vi "Delete Item.vi"(0 "State In":T1={"Prompt"="Click to add", "Listbox"=refnum, "Required"={"Strings"=[], "Bottom"=FALSE, "Italic"=FALSE, "FG"=0, "BG"=16777215, "Bold"=FALSE}, "Items"=[], "Req'd"=[], "Events"={"Items Changed"=refnum, "List Changed"=refnum}, "Max Rows"=-1, "Default name"=""}, 7 "Delete at":i32) -> (4 "State Out":T1={"Prompt"="Click to add", "Listbox"=refnum, "Required"={"Strings"=[], "Bottom"=FALSE, "Italic"=FALSE, "FG"=0, "BG"=16777215, "Bold"=FALSE}, "Items"=[], "Req'd"=[], "Events"={"Items Changed"=refnum, "List Changed"=refnum}, "Max Rows"=-1, "Default name"=""})   [LabVIEW 2015, in "KListboxEx.xctl"]
uses:
  KListboxEx.xctl
  State.ctl
  Required.ctl
  Events.ctl
  Event Action.ctl
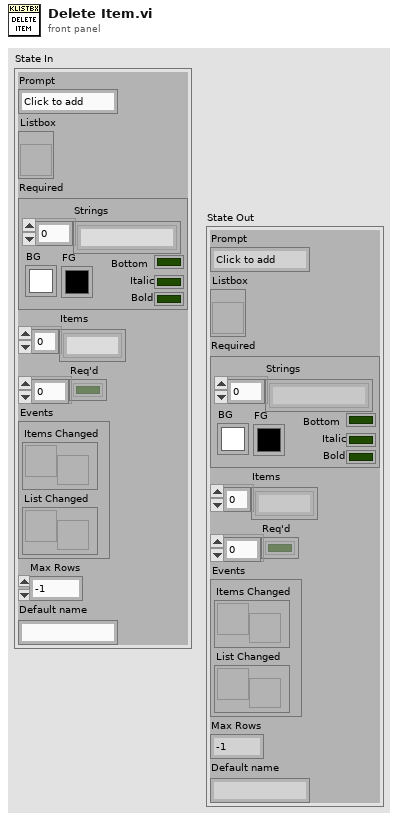
[diagram p1: front panel]
types:
  T1 = typedef "KListboxEx.xctl/State.ctl" = cluster{"Prompt":string, "Listbox":refnum<vi>, "Required":T2, "Items":string[], "Req'd":bool[], "Events":T3, "Max Rows":i32, "Default name":string}
  T2 = typedef "KListboxEx.xctl/Required.ctl" = cluster{"Strings":string[], "Bottom":bool, "Italic":bool, "FG":u32, "BG":u32, "Bold":bool}
  T3 = typedef "KListboxEx.xctl/Events.ctl" = cluster{"Items Changed":refnum<user-event>, "List Changed":refnum<user-event>}
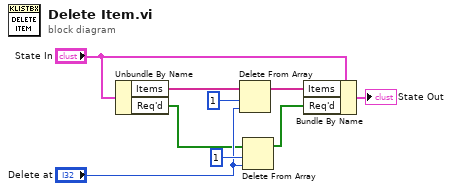
[diagram p0: block diagram]
diagram:
  n1 = Unbundle By Name("State In") -> ("Items"=w7:string[], "Req'd"=w3:bool[])
  n2 = Delete From Array(array=w7, length=1, index="Delete at") -> (array with subset deleted=w2:string[])  [unwired: 1 out]
  n3 = Delete From Array(array=w3, length=1, index="Delete at") -> (array with subset deleted=w1:bool[])  [unwired: 1 out]
  n4 = Bundle By Name(cluster="State In", "Items"=w2, "Req'd"=w1) -> (→"State Out":T1)
